vi "Begin.vi"(8 "error in":errorcluster) -> (0 "error out":errorcluster, 2 "pt cluster out":T1={"linear acuator left"={"DeviceStatus"={"status"=FALSE, "code"=0, "source"=""}, "Type"=enum."PWM", "PWM"={"PWM Channel"=enum."Invalid", "DeadBand"={"Name"="", "maxPositivePwm"=0, "minPositivePwm"=0, "centerPwm"=0, "maxNegativePwm"=0, "minNegativePwm"=0, "angularRange"=0}}, "CAN"={"Device Number"=0, "SetOutput VI Ref"=variant(refnum<vi> refnum), "GetOutput VI Ref"=variant(refnum<vi> refnum), "Enable VI Ref"=variant(refnum<vi> refnum), "Disable VI Ref"=variant(refnum<vi> refnum), "Data"=variant}, "Invert"=FALSE, "DIO PWM"={"PWM \"Enable\" Channel"=enum."Invalid", "DIOChannel"=enum."Invalid", "PWM Rate"=0.0}}, "arm extension"={"DeviceStatus"={"status"=FALSE, "code"=0, "source"=""}, "Type"=enum."PWM", "PWM"={"PWM Channel"=enum."Invalid", "DeadBand"={"Name"="", "maxPositivePwm"=0, "minPositivePwm"=0, "centerPwm"=0, "maxNegativePwm"=0, "minNegativePwm"=0, "angularRange"=0}}, "CAN"={"Device Number"=0, "SetOutput VI Ref"=variant(refnum<vi> refnum), "GetOutput VI Ref"=variant(refnum<vi> refnum), "Enable VI Ref"=variant(refnum<vi> refnum), "Disable VI Ref"=variant(refnum<vi> refnum), "Data"=variant}, "Invert"=FALSE, "DIO PWM"={"PWM \"Enable\" Channel"=enum."Invalid", "DIOChannel"=enum."Invalid", "PWM Rate"=0.0}}, "turret"={"DeviceStatus"={"status"=FALSE, "code"=0, "source"=""}, "Type"=enum."PWM", "PWM"={"PWM Channel"=enum."Invalid", "DeadBand"={"Name"="", "maxPositivePwm"=0, "minPositivePwm"=0, "centerPwm"=0, "maxNegativePwm"=0, "minNegativePwm"=0, "angularRange"=0}}, "CAN"={"Device Number"=0, "SetOutput VI Ref"=variant(refnum<vi> refnum), "GetOutput VI Ref"=variant(refnum<vi> refnum), "Enable VI Ref"=variant(refnum<vi> refnum), "Disable VI Ref"=variant(refnum<vi> refnum), "Data"=variant}, "Invert"=FALSE, "DIO PWM"={"PWM \"Enable\" Channel"=enum."Invalid", "DIOChannel"=enum."Invalid", "PWM Rate"=0.0}}, "hood"={"DeviceStatus"={"status"=FALSE, "code"=0, "source"=""}, "Type"=enum."PWM", "PWM"={"PWM Channel"=enum."Invalid", "DeadBand"={"Name"="", "maxPositivePwm"=0, "minPositivePwm"=0, "centerPwm"=0, "maxNegativePwm"=0, "minNegativePwm"=0, "angularRange"=0}}, "CAN"={"Device Number"=0, "SetOutput VI Ref"=variant(refnum<vi> refnum), "GetOutput VI Ref"=variant(refnum<vi> refnum), "Enable VI Ref"=variant(refnum<vi> refnum), "Disable VI Ref"=variant(refnum<vi> refnum), "Data"=variant}, "Invert"=FALSE, "DIO PWM"={"PWM \"Enable\" Channel"=enum."Invalid", "DIOChannel"=enum."Invalid", "PWM Rate"=0.0}}, "climb brake"={"DevStatus"={"status"=FALSE, "code"=0, "source"=""}, "Pneumatics Control Module"=0, "Forward Solenoid Channel"=enum."Solenoid 1", "Reverse Solenoid Channel"=enum."Invalid"}, "buddy climb"={"DevStatus"={"status"=FALSE, "code"=0, "source"=""}, "Pneumatics Control Module"=0, "Forward Solenoid Channel"=enum."Solenoid 1", "Reverse Solenoid Channel"=enum."Invalid"}, "drivetrain shifter"={"DevStatus"={"status"=FALSE, "code"=0, "source"=""}, "Pneumatics Control Module"=0, "Forward Solenoid Channel"=enum."Solenoid 1", "Reverse Solenoid Channel"=enum."Invalid"}, "hood"={"DevStatus"={"status"=FALSE, "code"=0, "source"=""}, "Pneumatics Control Module"=0, "Forward Solenoid Channel"=enum."Solenoid 1", "Reverse Solenoid Channel"=enum."Invalid"}, "climber encoder"={"DevStatus"={"status"=FALSE, "code"=0, "source"=""}, "EncoderIndex"=enum."Enc 0", "CounterIndex"=enum."Ctr 0", "DistancePerCount"=1.0, "Decoding Type"=enum."4x"}, "shooter encoder"={"DevStatus"={"status"=FALSE, "code"=0, "source"=""}, "EncoderIndex"=enum."Enc 0", "CounterIndex"=enum."Ctr 0", "DistancePerCount"=1.0, "Decoding Type"=enum."4x"}, "color sensor"={"I2CDevRef"={"DevStatus"={"status"=FALSE, "code"=0, "source"=""}, "Device Address"=0, "Handle"=0, "I2C Bus"=enum."Invalid"}}, "linear acuator left pot"={"DevStatus"={"status"=FALSE, "code"=0, "source"=""}, "Analog Channel"=enum."Invalid", "Invert Output"=FALSE}, "linear acuator right pot "={"DevStatus"={"status"=FALSE, "code"=0, "source"=""}, "Analog Channel"=enum."Invalid", "Invert Output"=FALSE}, "auto balancer pot"={"DevStatus"={"status"=FALSE, "code"=0, "source"=""}, "Analog Channel"=enum."Invalid", "Invert Output"=FALSE}, "shooter"={"DeviceStatus"={"status"=FALSE, "code"=0, "source"=""}, "Type"=enum."PWM", "PWM"={"PWM Channel"=enum."Invalid", "DeadBand"={"Name"="", "maxPositivePwm"=0, "minPositivePwm"=0, "centerPwm"=0, "maxNegativePwm"=0, "minNegativePwm"=0, "angularRange"=0}}, "CAN"={"Device Number"=0, "SetOutput VI Ref"=variant(refnum<vi> refnum), "GetOutput VI Ref"=variant(refnum<vi> refnum), "Enable VI Ref"=variant(refnum<vi> refnum), "Disable VI Ref"=variant(refnum<vi> refnum), "Data"=variant}, "Invert"=FALSE, "DIO PWM"={"PWM \"Enable\" Channel"=enum."Invalid", "DIOChannel"=enum."Invalid", "PWM Rate"=0.0}}, "hopper"={"DeviceStatus"={"status"=FALSE, "code"=0, "source"=""}, "Type"=enum."PWM", "PWM"={"PWM Channel"=enum."Invalid", "DeadBand"={"Name"="", "maxPositivePwm"=0, "minPositivePwm"=0, "centerPwm"=0, "maxNegativePwm"=0, "minNegativePwm"=0, "angularRange"=0}}, "CAN"={"Device Number"=0, "SetOutput VI Ref"=variant(refnum<vi> refnum), "GetOutput VI Ref"=variant(refnum<vi> refnum), "Enable VI Ref"=variant(refnum<vi> refnum), "Disable VI Ref"=variant(refnum<vi> refnum), "Data"=variant}, "Invert"=FALSE, "DIO PWM"={"PWM \"Enable\" Channel"=enum."Invalid", "DIOChannel"=enum."Invalid", "PWM Rate"=0.0}}, "feeder"={"DeviceStatus"={"status"=FALSE, "code"=0, "source"=""}, "Type"=enum."PWM", "PWM"={"PWM Channel"=enum."Invalid", "DeadBand"={"Name"="", "maxPositivePwm"=0, "minPositivePwm"=0, "centerPwm"=0, "maxNegativePwm"=0, "minNegativePwm"=0, "angularRange"=0}}, "CAN"={"Device Number"=0, "SetOutput VI Ref"=variant(refnum<vi> refnum), "GetOutput VI Ref"=variant(refnum<vi> refnum), "Enable VI Ref"=variant(refnum<vi> refnum), "Disable VI Ref"=variant(refnum<vi> refnum), "Data"=variant}, "Invert"=FALSE, "DIO PWM"={"PWM \"Enable\" Channel"=enum."Invalid", "DIOChannel"=enum."Invalid", "PWM Rate"=0.0}}, "intake"={"DeviceStatus"={"status"=FALSE, "code"=0, "source"=""}, "Type"=enum."PWM", "PWM"={"PWM Channel"=enum."Invalid", "DeadBand"={"Name"="", "maxPositivePwm"=0, "minPositivePwm"=0, "centerPwm"=0, "maxNegativePwm"=0, "minNegativePwm"=0, "angularRange"=0}}, "CAN"={"Device Number"=0, "SetOutput VI Ref"=variant(refnum<vi> refnum), "GetOutput VI Ref"=variant(refnum<vi> refnum), "Enable VI Ref"=variant(refnum<vi> refnum), "Disable VI Ref"=variant(refnum<vi> refnum), "Data"=variant}, "Invert"=FALSE, "DIO PWM"={"PWM \"Enable\" Channel"=enum."Invalid", "DIOChannel"=enum."Invalid", "PWM Rate"=0.0}}, "auto balance"={"DeviceStatus"={"status"=FALSE, "code"=0, "source"=""}, "Type"=enum."PWM", "PWM"={"PWM Channel"=enum."Invalid", "DeadBand"={"Name"="", "maxPositivePwm"=0, "minPositivePwm"=0, "centerPwm"=0, "maxNegativePwm"=0, "minNegativePwm"=0, "angularRange"=0}}, "CAN"={"Device Number"=0, "SetOutput VI Ref"=variant(refnum<vi> refnum), "GetOutput VI Ref"=variant(refnum<vi> refnum), "Enable VI Ref"=variant(refnum<vi> refnum), "Disable VI Ref"=variant(refnum<vi> refnum), "Data"=variant}, "Invert"=FALSE, "DIO PWM"={"PWM \"Enable\" Channel"=enum."Invalid", "DIOChannel"=enum."Invalid", "PWM Rate"=0.0}}, "linear acuator right"={"DeviceStatus"={"status"=FALSE, "code"=0, "source"=""}, "Type"=enum."PWM", "PWM"={"PWM Channel"=enum."Invalid", "DeadBand"={"Name"="", "maxPositivePwm"=0, "minPositivePwm"=0, "centerPwm"=0, "maxNegativePwm"=0, "minNegativePwm"=0, "angularRange"=0}}, "CAN"={"Device Number"=0, "SetOutput VI Ref"=variant(refnum<vi> refnum), "GetOutput VI Ref"=variant(refnum<vi> refnum), "Enable VI Ref"=variant(refnum<vi> refnum), "Disable VI Ref"=variant(refnum<vi> refnum), "Data"=variant}, "Invert"=FALSE, "DIO PWM"={"PWM \"Enable\" Channel"=enum."Invalid", "DIOChannel"=enum."Invalid", "PWM Rate"=0.0}}} {"color sensor"."I2CDevRef"."Device Address" format="%.0x"}, 3 "Teleop/Auto Cluster Out":T18={"x Joystick"={"Device"=enum."USB 1"}, "y Joystick"={"Device"=enum."USB 1"}, "controller"={"Device"=enum."USB 1"}, "right drive encoder"={"DevStatus"={"status"=FALSE, "code"=0, "source"=""}, "EncoderIndex"=enum."Enc 0", "CounterIndex"=enum."Ctr 0", "DistancePerCount"=1.0, "Decoding Type"=enum."4x"}, "left drive encoder"={"DevStatus"={"status"=FALSE, "code"=0, "source"=""}, "EncoderIndex"=enum."Enc 0", "CounterIndex"=enum."Ctr 0", "DistancePerCount"=1.0, "Decoding Type"=enum."4x"}, "drive motors"={"DevStatus"={"status"=FALSE, "code"=0, "source"=""}, "Motors[]"=[], "Square Inputs"=FALSE, "Max Output"=1.0}, "gyro"={"DeviceStatus"={"status"=FALSE, "code"=0, "source"=""}, "Device Number"=0, "Type"=352321536, "Device ID"=0, "Handle"=0, "UsageFrame"=0, "Library Path"=path ""}, "drive buttons"={"Device"=enum."USB 1"}} {"gyro"."Type" items=["CAN"=352321536, "TalonSRX"=33554432]})   [LabVIEW 2019]
doc: "Called before other user functions, this VI is expected to open initial I/O refnums, load in file data, and do all program initialization. Notice that the <B>error out</B> terminal is simply used for data flow. Wiring it to other structures or subVIs ensures that this VI runs first."
uses:
  <vilib>/Rock Robotics/WPI/RobotDrive/WPI_RobotDriveDevRef.ctl
  <vilib>/Rock Robotics/WPI/MotorControl/WPI_MotorControlDeviceRef.ctl
  <vilib>/Rock Robotics/WPI/MotorControl/WPI_MotorControlType.ctl
  <vilib>/Rock Robotics/SystemInterfaces/DIO/FPGA_DIOPWMChannel.ctl
  <vilib>/Rock Robotics/WPI/PWM/WPI_PWMDeadband.ctl
  <vilib>/Rock Robotics/SystemInterfaces/DIO/FPGA_DIOChannel.ctl
  teleop auto cluster.ctl
  <vilib>/Rock Robotics/WPI/Joystick/WPI_JoystickDevRef.ctl
  <vilib>/Rock Robotics/WPI/Joystick/WPI_JoystickDeviceEnum.ctl
  <vilib>/Rock Robotics/WPI/Encoder/WPI_EncoderDevRef.ctl
  <vilib>/Rock Robotics/SystemInterfaces/Encoder/FPGA_EncoderIdx.ctl
  <vilib>/Rock Robotics/SystemInterfaces/Counter/FPGA_CounterCtrSystemIndex.ctl
  <vilib>/Rock Robotics/WPI/Encoder/WPI_EncoderType.ctl
  <vilib>/Rock Robotics/WPI/ThirdParty/Phoenix-LabVIEW/Pigeon IMU/CTRE_PigeonIMU_DeviceRef.ctl
  <vilib>/Rock Robotics/WPI/ThirdParty/Phoenix-LabVIEW/Pigeon IMU/CTRE_PigeonIMU_ConnectionType.ctl
  ptclustergood.ctl
  <vilib>/Rock Robotics/WPI/Solenoid/WPI_SolenoidDevRef.ctl
  <vilib>/Rock Robotics/WPI/Solenoid/WPI_SolenoidChannel.ctl
  <vilib>/Rock Robotics/WPI/ThirdParty/REV Robotics/Color SensorV3/Typedef/Color Sensor V3 DevRef.ctl
  <vilib>/Rock Robotics/WPI/I2C/WPI_I2CDevRef.ctl
  <vilib>/Rock Robotics/SystemInterfaces/i2clib/i2c_bus.ctl
  <vilib>/Rock Robotics/WPI/Potentiometer/WPI_PotentiometerDevRef.ctl
  <vilib>/Rock Robotics/SystemInterfaces/AI/FPGA_AIChannel.ctl
  <vilib>/Rock Robotics/WPI/DriverStation/WPI_DriverStationRobotMode2.ctl
  <vilib>/Rock Robotics/WPI/Solenoid/WPI_SolenoidValue.ctl
  <vilib>/Rock Robotics/WPI/ThirdParty/Phoenix-LabVIEW/Pigeon IMU/CTRE_PigeonIMU_TareType.ctl
  Robot Global Data.vi
  <vilib>/Rock Robotics/WPI/Counter/WPI_CounterDigitalInputToDigitalSource.vi
  <vilib>/Rock Robotics/WPI/Solenoid/WPI_SolenoidOpenDouble.vi
  <vilib>/Rock Robotics/WPI/Solenoid/WPI_SolenoidSetEnum.vi
  <vilib>/Rock Robotics/WPI/ThirdParty/Phoenix-LabVIEW/Pigeon IMU/CTRE_PigeonIMU_Open_CAN.vi
  GlobalVariables.vi
panel:
  in  "pt cluster":T1={"linear acuator left"={"DeviceStatus"={"status"=FALSE, "code"=0, "source"=""}, "Type"=enum."PWM", "PWM"={"PWM Channel"=enum."Invalid", "DeadBand"={"Name"="", "maxPositivePwm"=0, "minPositivePwm"=0, "centerPwm"=0, "maxNegativePwm"=0, "minNegativePwm"=0, "angularRange"=0}}, "CAN"={"Device Number"=0, "SetOutput VI Ref"=variant(refnum<vi> refnum), "GetOutput VI Ref"=variant(refnum<vi> refnum), "Enable VI Ref"=variant(refnum<vi> refnum), "Disable VI Ref"=variant(refnum<vi> refnum), "Data"=variant}, "Invert"=FALSE, "DIO PWM"={"PWM \"Enable\" Channel"=enum."Invalid", "DIOChannel"=enum."Invalid", "PWM Rate"=0.0}}, "arm extension"={"DeviceStatus"={"status"=FALSE, "code"=0, "source"=""}, "Type"=enum."PWM", "PWM"={"PWM Channel"=enum."Invalid", "DeadBand"={"Name"="", "maxPositivePwm"=0, "minPositivePwm"=0, "centerPwm"=0, "maxNegativePwm"=0, "minNegativePwm"=0, "angularRange"=0}}, "CAN"={"Device Number"=0, "SetOutput VI Ref"=variant(refnum<vi> refnum), "GetOutput VI Ref"=variant(refnum<vi> refnum), "Enable VI Ref"=variant(refnum<vi> refnum), "Disable VI Ref"=variant(refnum<vi> refnum), "Data"=variant}, "Invert"=FALSE, "DIO PWM"={"PWM \"Enable\" Channel"=enum."Invalid", "DIOChannel"=enum."Invalid", "PWM Rate"=0.0}}, "turret"={"DeviceStatus"={"status"=FALSE, "code"=0, "source"=""}, "Type"=enum."PWM", "PWM"={"PWM Channel"=enum."Invalid", "DeadBand"={"Name"="", "maxPositivePwm"=0, "minPositivePwm"=0, "centerPwm"=0, "maxNegativePwm"=0, "minNegativePwm"=0, "angularRange"=0}}, "CAN"={"Device Number"=0, "SetOutput VI Ref"=variant(refnum<vi> refnum), "GetOutput VI Ref"=variant(refnum<vi> refnum), "Enable VI Ref"=variant(refnum<vi> refnum), "Disable VI Ref"=variant(refnum<vi> refnum), "Data"=variant}, "Invert"=FALSE, "DIO PWM"={"PWM \"Enable\" Channel"=enum."Invalid", "DIOChannel"=enum."Invalid", "PWM Rate"=0.0}}, "hood"={"DeviceStatus"={"status"=FALSE, "code"=0, "source"=""}, "Type"=enum."PWM", "PWM"={"PWM Channel"=enum."Invalid", "DeadBand"={"Name"="", "maxPositivePwm"=0, "minPositivePwm"=0, "centerPwm"=0, "maxNegativePwm"=0, "minNegativePwm"=0, "angularRange"=0}}, "CAN"={"Device Number"=0, "SetOutput VI Ref"=variant(refnum<vi> refnum), "GetOutput VI Ref"=variant(refnum<vi> refnum), "Enable VI Ref"=variant(refnum<vi> refnum), "Disable VI Ref"=variant(refnum<vi> refnum), "Data"=variant}, "Invert"=FALSE, "DIO PWM"={"PWM \"Enable\" Channel"=enum."Invalid", "DIOChannel"=enum."Invalid", "PWM Rate"=0.0}}, "climb brake"={"DevStatus"={"status"=FALSE, "code"=0, "source"=""}, "Pneumatics Control Module"=0, "Forward Solenoid Channel"=enum."Solenoid 1", "Reverse Solenoid Channel"=enum."Invalid"}, "buddy climb"={"DevStatus"={"status"=FALSE, "code"=0, "source"=""}, "Pneumatics Control Module"=0, "Forward Solenoid Channel"=enum."Solenoid 1", "Reverse Solenoid Channel"=enum."Invalid"}, "drivetrain shifter"={"DevStatus"={"status"=FALSE, "code"=0, "source"=""}, "Pneumatics Control Module"=0, "Forward Solenoid Channel"=enum."Solenoid 1", "Reverse Solenoid Channel"=enum."Invalid"}, "hood"={"DevStatus"={"status"=FALSE, "code"=0, "source"=""}, "Pneumatics Control Module"=0, "Forward Solenoid Channel"=enum."Solenoid 1", "Reverse Solenoid Channel"=enum."Invalid"}, "climber encoder"={"DevStatus"={"status"=FALSE, "code"=0, "source"=""}, "EncoderIndex"=enum."Enc 0", "CounterIndex"=enum."Ctr 0", "DistancePerCount"=1.0, "Decoding Type"=enum."4x"}, "shooter encoder"={"DevStatus"={"status"=FALSE, "code"=0, "source"=""}, "EncoderIndex"=enum."Enc 0", "CounterIndex"=enum."Ctr 0", "DistancePerCount"=1.0, "Decoding Type"=enum."4x"}, "color sensor"={"I2CDevRef"={"DevStatus"={"status"=FALSE, "code"=0, "source"=""}, "Device Address"=0, "Handle"=0, "I2C Bus"=enum."Invalid"}}, "linear acuator left pot"={"DevStatus"={"status"=FALSE, "code"=0, "source"=""}, "Analog Channel"=enum."Invalid", "Invert Output"=FALSE}, "linear acuator right pot "={"DevStatus"={"status"=FALSE, "code"=0, "source"=""}, "Analog Channel"=enum."Invalid", "Invert Output"=FALSE}, "auto balancer pot"={"DevStatus"={"status"=FALSE, "code"=0, "source"=""}, "Analog Channel"=enum."Invalid", "Invert Output"=FALSE}, "shooter"={"DeviceStatus"={"status"=FALSE, "code"=0, "source"=""}, "Type"=enum."PWM", "PWM"={"PWM Channel"=enum."Invalid", "DeadBand"={"Name"="", "maxPositivePwm"=0, "minPositivePwm"=0, "centerPwm"=0, "maxNegativePwm"=0, "minNegativePwm"=0, "angularRange"=0}}, "CAN"={"Device Number"=0, "SetOutput VI Ref"=variant(refnum<vi> refnum), "GetOutput VI Ref"=variant(refnum<vi> refnum), "Enable VI Ref"=variant(refnum<vi> refnum), "Disable VI Ref"=variant(refnum<vi> refnum), "Data"=variant}, "Invert"=FALSE, "DIO PWM"={"PWM \"Enable\" Channel"=enum."Invalid", "DIOChannel"=enum."Invalid", "PWM Rate"=0.0}}, "hopper"={"DeviceStatus"={"status"=FALSE, "code"=0, "source"=""}, "Type"=enum."PWM", "PWM"={"PWM Channel"=enum."Invalid", "DeadBand"={"Name"="", "maxPositivePwm"=0, "minPositivePwm"=0, "centerPwm"=0, "maxNegativePwm"=0, "minNegativePwm"=0, "angularRange"=0}}, "CAN"={"Device Number"=0, "SetOutput VI Ref"=variant(refnum<vi> refnum), "GetOutput VI Ref"=variant(refnum<vi> refnum), "Enable VI Ref"=variant(refnum<vi> refnum), "Disable VI Ref"=variant(refnum<vi> refnum), "Data"=variant}, "Invert"=FALSE, "DIO PWM"={"PWM \"Enable\" Channel"=enum."Invalid", "DIOChannel"=enum."Invalid", "PWM Rate"=0.0}}, "feeder"={"DeviceStatus"={"status"=FALSE, "code"=0, "source"=""}, "Type"=enum."PWM", "PWM"={"PWM Channel"=enum."Invalid", "DeadBand"={"Name"="", "maxPositivePwm"=0, "minPositivePwm"=0, "centerPwm"=0, "maxNegativePwm"=0, "minNegativePwm"=0, "angularRange"=0}}, "CAN"={"Device Number"=0, "SetOutput VI Ref"=variant(refnum<vi> refnum), "GetOutput VI Ref"=variant(refnum<vi> refnum), "Enable VI Ref"=variant(refnum<vi> refnum), "Disable VI Ref"=variant(refnum<vi> refnum), "Data"=variant}, "Invert"=FALSE, "DIO PWM"={"PWM \"Enable\" Channel"=enum."Invalid", "DIOChannel"=enum."Invalid", "PWM Rate"=0.0}}, "intake"={"DeviceStatus"={"status"=FALSE, "code"=0, "source"=""}, "Type"=enum."PWM", "PWM"={"PWM Channel"=enum."Invalid", "DeadBand"={"Name"="", "maxPositivePwm"=0, "minPositivePwm"=0, "centerPwm"=0, "maxNegativePwm"=0, "minNegativePwm"=0, "angularRange"=0}}, "CAN"={"Device Number"=0, "SetOutput VI Ref"=variant(refnum<vi> refnum), "GetOutput VI Ref"=variant(refnum<vi> refnum), "Enable VI Ref"=variant(refnum<vi> refnum), "Disable VI Ref"=variant(refnum<vi> refnum), "Data"=variant}, "Invert"=FALSE, "DIO PWM"={"PWM \"Enable\" Channel"=enum."Invalid", "DIOChannel"=enum."Invalid", "PWM Rate"=0.0}}, "auto balance"={"DeviceStatus"={"status"=FALSE, "code"=0, "source"=""}, "Type"=enum."PWM", "PWM"={"PWM Channel"=enum."Invalid", "DeadBand"={"Name"="", "maxPositivePwm"=0, "minPositivePwm"=0, "centerPwm"=0, "maxNegativePwm"=0, "minNegativePwm"=0, "angularRange"=0}}, "CAN"={"Device Number"=0, "SetOutput VI Ref"=variant(refnum<vi> refnum), "GetOutput VI Ref"=variant(refnum<vi> refnum), "Enable VI Ref"=variant(refnum<vi> refnum), "Disable VI Ref"=variant(refnum<vi> refnum), "Data"=variant}, "Invert"=FALSE, "DIO PWM"={"PWM \"Enable\" Channel"=enum."Invalid", "DIOChannel"=enum."Invalid", "PWM Rate"=0.0}}, "linear acuator right"={"DeviceStatus"={"status"=FALSE, "code"=0, "source"=""}, "Type"=enum."PWM", "PWM"={"PWM Channel"=enum."Invalid", "DeadBand"={"Name"="", "maxPositivePwm"=0, "minPositivePwm"=0, "centerPwm"=0, "maxNegativePwm"=0, "minNegativePwm"=0, "angularRange"=0}}, "CAN"={"Device Number"=0, "SetOutput VI Ref"=variant(refnum<vi> refnum), "GetOutput VI Ref"=variant(refnum<vi> refnum), "Enable VI Ref"=variant(refnum<vi> refnum), "Disable VI Ref"=variant(refnum<vi> refnum), "Data"=variant}, "Invert"=FALSE, "DIO PWM"={"PWM \"Enable\" Channel"=enum."Invalid", "DIOChannel"=enum."Invalid", "PWM Rate"=0.0}}} {"color sensor"."I2CDevRef"."Device Address" format="%.0x"}
  in  "Teleop/Auto Cluster":T18={"x Joystick"={"Device"=enum."USB 1"}, "y Joystick"={"Device"=enum."USB 1"}, "controller"={"Device"=enum."USB 1"}, "right drive encoder"={"DevStatus"={"status"=FALSE, "code"=0, "source"=""}, "EncoderIndex"=enum."Enc 0", "CounterIndex"=enum."Ctr 0", "DistancePerCount"=1.0, "Decoding Type"=enum."4x"}, "left drive encoder"={"DevStatus"={"status"=FALSE, "code"=0, "source"=""}, "EncoderIndex"=enum."Enc 0", "CounterIndex"=enum."Ctr 0", "DistancePerCount"=1.0, "Decoding Type"=enum."4x"}, "drive motors"={"DevStatus"={"status"=FALSE, "code"=0, "source"=""}, "Motors[]"=[], "Square Inputs"=FALSE, "Max Output"=1.0}, "gyro"={"DeviceStatus"={"status"=FALSE, "code"=0, "source"=""}, "Device Number"=0, "Type"=352321536, "Device ID"=0, "Handle"=0, "UsageFrame"=0, "Library Path"=path ""}, "drive buttons"={"Device"=enum."USB 1"}} {"gyro"."Type" items=["CAN"=352321536, "TalonSRX"=33554432]}
  in  "RobotDriveDevRef":T21={"DevStatus"={"status"=FALSE, "code"=0, "source"=""}, "Motors[]"=[], "Square Inputs"=FALSE, "Max Output"=1.0}
  in  "DevStatus":errorcluster
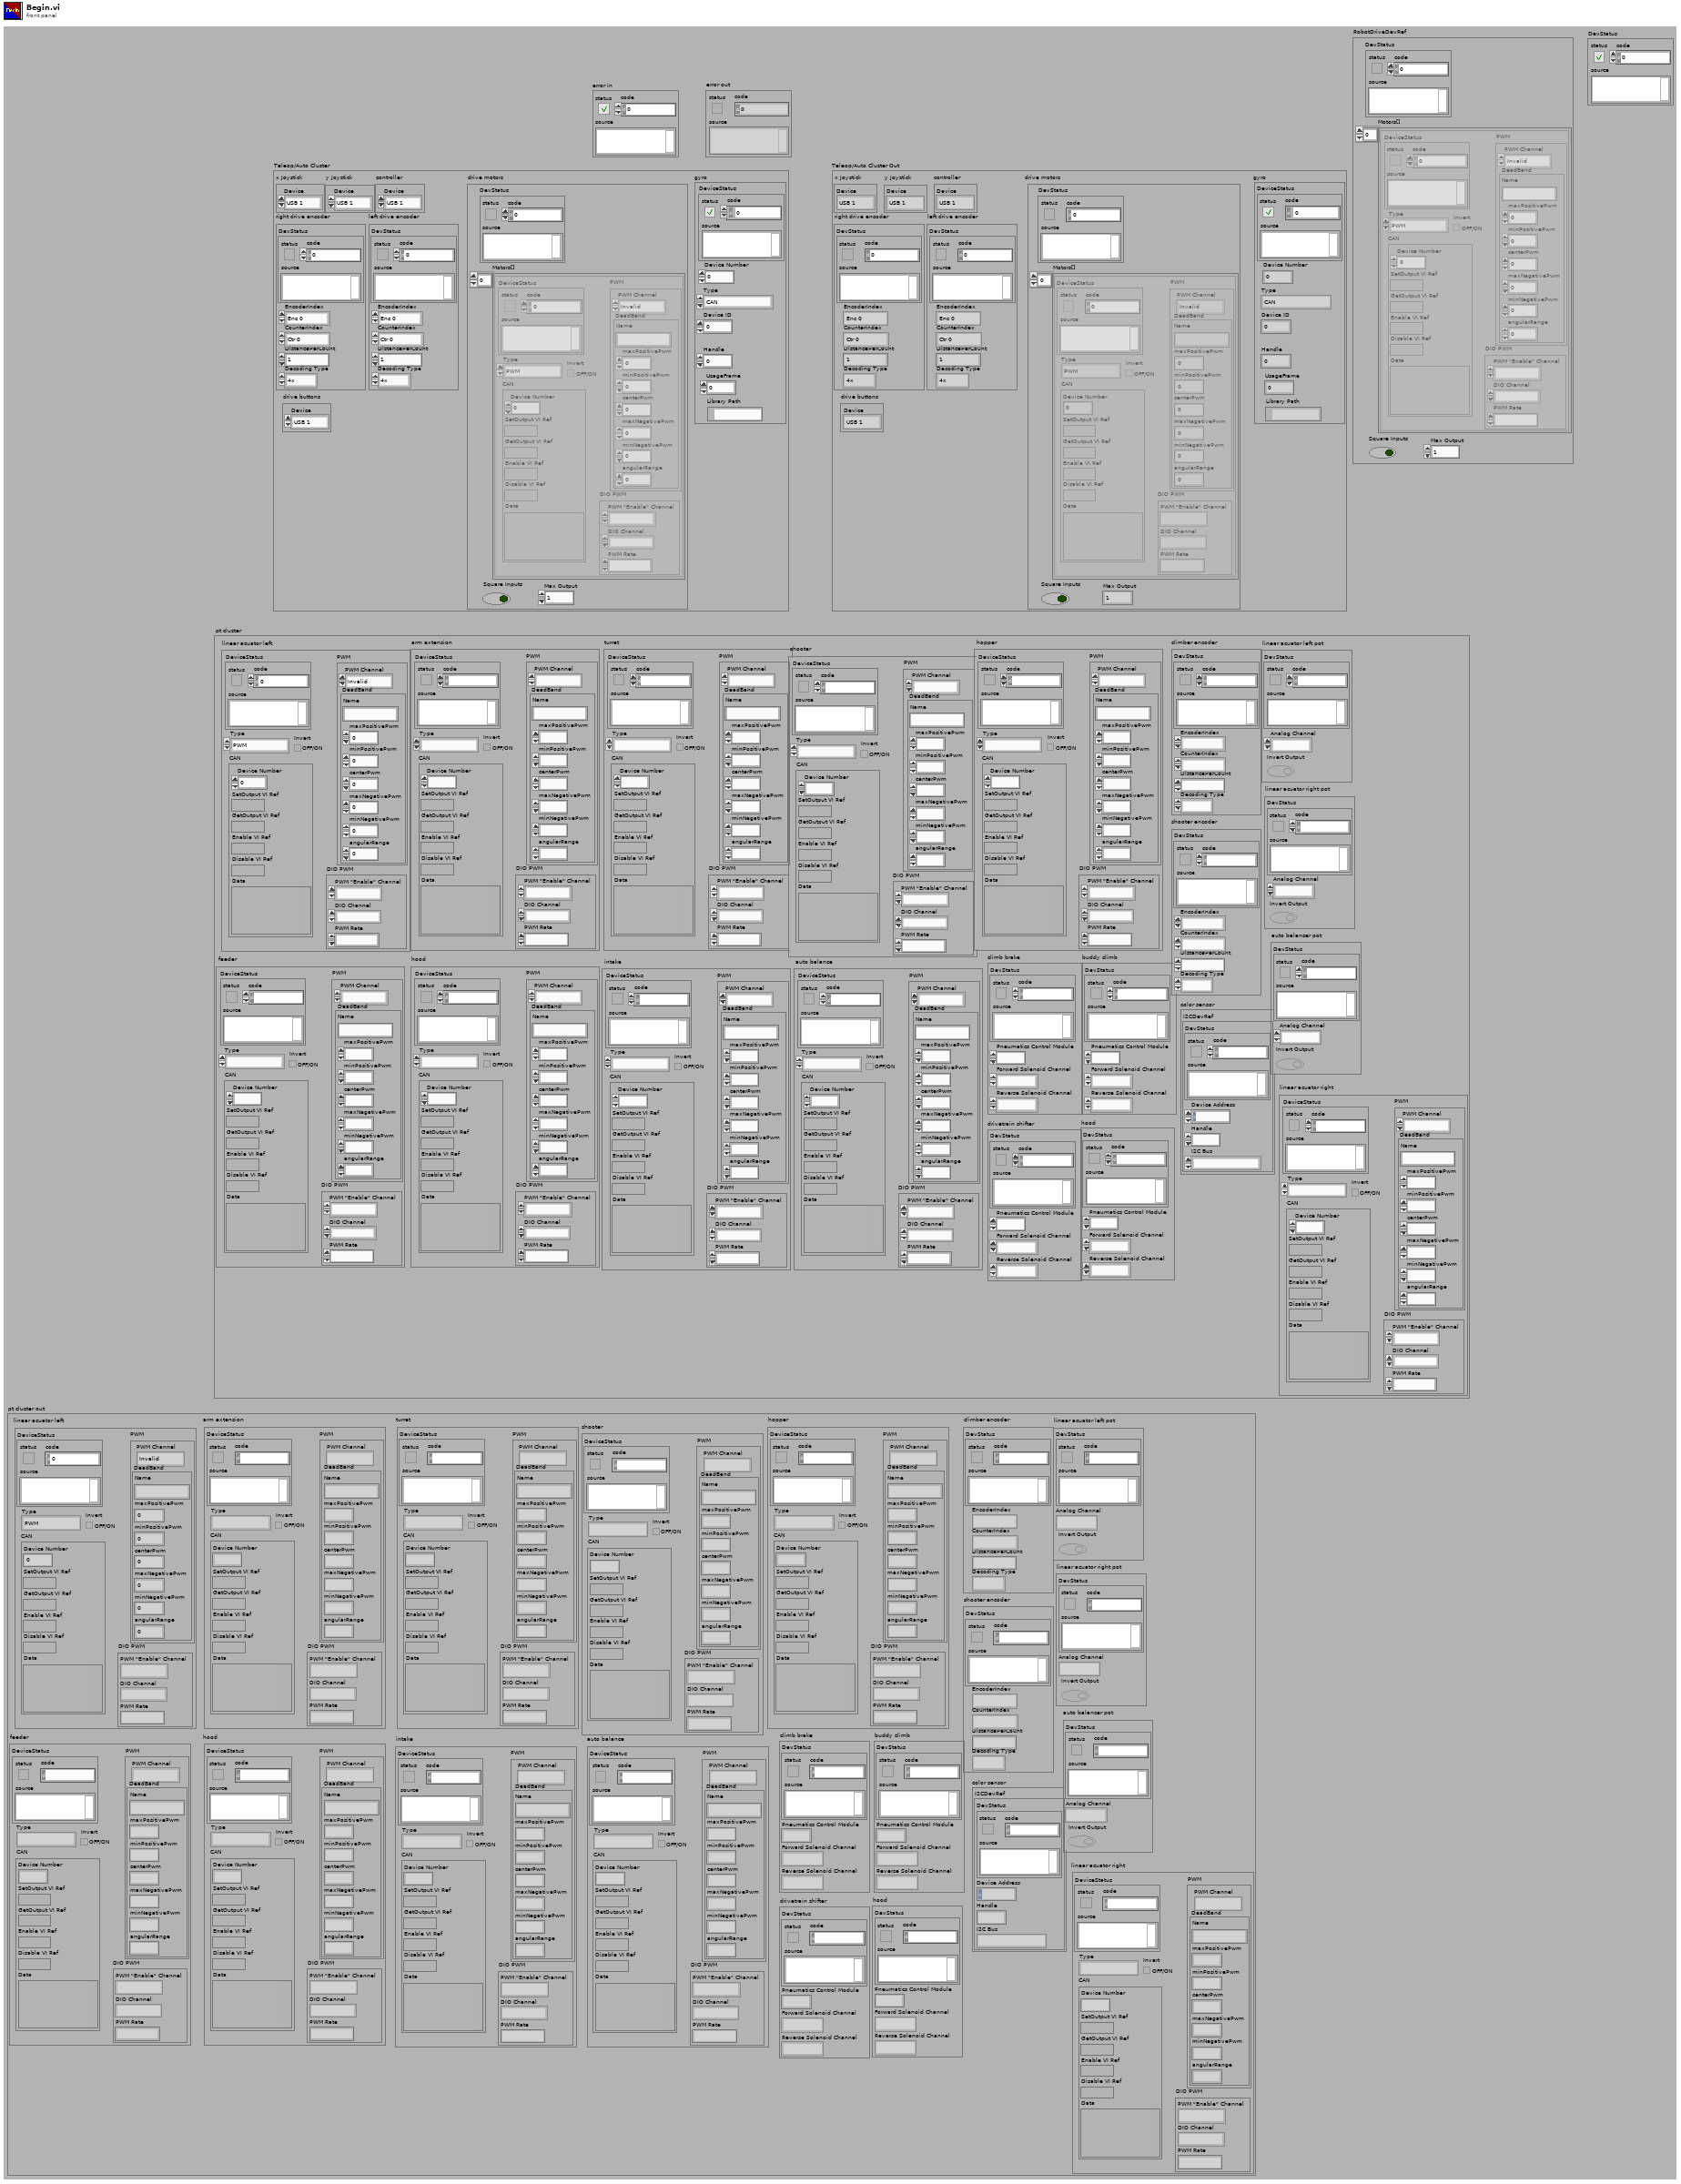
[diagram p1: front panel]
types:
  T1 = typedef "ptclustergood.ctl" = cluster{"linear acuator left":T2, "arm extension":T2, "turret":T2, "hood":T2, "climb brake":T7, "buddy climb":T7, "drivetrain shifter":T7, "hood":T7, "climber encoder":T9, "shooter encoder":T9, "color sensor":T13, "linear acuator left pot":T16, "linear acuator right pot ":T16, "auto balancer pot":T16, "shooter":T2, "hopper":T2, "feeder":T2, "intake":T2, "auto balance":T2, "linear acuator right":T2}
  T2 = typedef "WPI_MotorControlDeviceRef.ctl" = cluster{"DeviceStatus":errorcluster, "Type":T3, "PWM":cluster{"PWM Channel":T4, "DeadBand":T5}, "CAN":cluster{"Device Number":u8, "SetOutput VI Ref":variant, "GetOutput VI Ref":variant, "Enable VI Ref":variant, "Disable VI Ref":variant, "Data":variant}, "Invert":bool, "DIO PWM":cluster{"PWM \"Enable\" Channel":T4, "DIOChannel":T6, "PWM Rate":dbl}}
  T3 = typedef "WPI_MotorControlType.ctl" = enum16{"PWM", "CAN", "DIO PWM"}
  T4 = typedef "FPGA_DIOPWMChannel.ctl" = enum8{"PWM 0", "PWM 1", "PWM 2", "PWM 3", "PWM 4", "PWM 5", "PWM 6", "PWM 7", "PWM 8", "PWM 9", "PWM MXP 0", "PWM MXP 1", "PWM MXP 2", "PWM MXP 3", "PWM MXP 4", "PWM MXP 5", "PWM MXP 6", "PWM MXP 7", "PWM MXP 8", "PWM MXP 9", "Invalid"}
  T5 = typedef "WPI_PWMDeadband.ctl" = cluster{"Name":string, "maxPositivePwm":i32, "minPositivePwm":i32, "centerPwm":i32, "maxNegativePwm":i32, "minNegativePwm":i32, "angularRange":u16}
  T6 = typedef "FPGA_DIOChannel.ctl" = enum8{"DIO 0", "DIO 1", "DIO 2", "DIO 3", "DIO 4", "DIO 5", "DIO 6", "DIO 7", "DIO 8", "DIO 9", "DIO MXP 0", "DIO MXP 1", "DIO MXP 2", "DIO MXP 3", "DIO MXP 4", "DIO MXP 5", "DIO MXP 6", "DIO MXP 7", "DIO MXP 8", "DIO MXP 9", "DIO MXP 10", "DIO MXP 11", "DIO MXP 12", "DIO MXP 13", "DIO MXP 14", "DIO MXP 15", "SPI Port CS1", "SPI Port CS2", "SPI Port CS3", "SPI Port MISO", "SPI Port MOSI", "Invalid"}
  T7 = typedef "WPI_SolenoidDevRef.ctl" = cluster{"DevStatus":errorcluster, "Pneumatics Control Module":u8, "Forward Solenoid Channel":T8, "Reverse Solenoid Channel":T8}
  T8 = typedef "WPI_SolenoidChannel.ctl" = enum8{"Solenoid 0", "Solenoid 1", "Solenoid 2", "Solenoid 3", "Solenoid 4", "Solenoid 5", "Solenoid 6", "Solenoid 7", "Invalid"}
  T9 = typedef "WPI_EncoderDevRef.ctl" = cluster{"DevStatus":errorcluster, "EncoderIndex":T10, "CounterIndex":T11, "DistancePerCount":dbl, "Decoding Type":T12}
  T10 = typedef "FPGA_EncoderIdx.ctl" = enum8{"Enc 0", "Enc 1", "Enc 2", "Enc 3", "Enc 4", "Enc 5", "Enc 6", "Enc 7", "Invalid"}
  T11 = typedef "FPGA_CounterCtrSystemIndex.ctl" = enum8{"Ctr 0", "Ctr 1", "Ctr 2", "Ctr 3", "Ctr 4", "Ctr 5", "Ctr 6", "Ctr 7", "Invalid"}
  T12 = typedef "WPI_EncoderType.ctl" = enum16{"1x", "2x", "4x"}
  T13 = typedef "Color Sensor V3 DevRef.ctl" = cluster{"I2CDevRef":T14}
  T14 = typedef "WPI_I2CDevRef.ctl" = cluster{"DevStatus":errorcluster, "Device Address":u8, "Handle":i32, "I2C Bus":T15}
  T15 = typedef "i2c_bus.ctl" = enum16{"I2C On-Board", "I2C MXP", "Invalid"}
  T16 = typedef "WPI_PotentiometerDevRef.ctl" = cluster{"DevStatus":errorcluster, "Analog Channel":T17, "Invert Output":bool}
  T17 = typedef "FPGA_AIChannel.ctl" = enum8{"AI 0", "AI 1", "AI 2", "AI 3", "AI MXP 0", "AI MXP 1", "AI MXP 2", "AI MXP 3", "Invalid"}
  T18 = typedef "teleop auto cluster.ctl" = cluster{"x Joystick":T19, "y Joystick":T19, "controller":T19, "right drive encoder":T9, "left drive encoder":T9, "drive motors":T21, "gyro":T22, "drive buttons":T19}
  T19 = typedef "WPI_JoystickDevRef.ctl" = cluster{"Device":T20}
  T20 = typedef "WPI_JoystickDeviceEnum.ctl" = enum16{"USB 0", "USB 1", "USB 2", "USB 3", "USB 4", "USB 5"}
  T21 = typedef "WPI_RobotDriveDevRef.ctl" = cluster{"DevStatus":errorcluster, "Motors[]":T2[], "Square Inputs":bool, "Max Output":dbl}
  T22 = typedef "CTRE_PigeonIMU_DeviceRef.ctl" = cluster{"DeviceStatus":errorcluster, "Device Number":u8, "Type":T23, "Device ID":u32, "Handle":u64, "UsageFrame":u32, "Library Path":path}
  T23 = typedef "CTRE_PigeonIMU_ConnectionType.ctl" = u32
  T24 = enum16{"ground protect", "ground pickup", "control panel", "shooting", "climb", "unjam", "intake shoot"}
  T25 = typedef "WPI_SolenoidValue.ctl" = enum16{"Off", "On", "Forward", "Reverse"}
  T26 = typedef "CTRE_PigeonIMU_TareType.ctl" = u8
  T27 = typedef "WPI_DriverStationRobotMode2.ctl" = enum16{"Autonomous Disabled", "Autonomous Enabled", "Teleop Disabled", "Teleop Enabled", "Disconnected", "Finish", "Test Disabled", "Test Enabled", "Emergency Stopped"}
  T28 = typedef "WPI_DigitalInputDevRef.ctl" = cluster{"DevStatus":errorcluster, "DIO Channel":T6}
  T29 = typedef "FPGA_CounterEncoderSourceConvertionLVSourceType.ctl" = cluster{"DevStatus":errorcluster, "AnalogTriggerMode?":bool, "DigitalMode":cluster{"DIO Channel":T30}, "AnalogTriggerMode":cluster{"AnalogTriggerIndex":T31, "OutputType":T32}}
  T30 = typedef "FPGA_DIODigitalSourceChannel.ctl" = enum8{"DIO 0", "DIO 1", "DIO 2", "DIO 3", "DIO 4", "DIO 5", "DIO 6", "DIO 7", "DIO 8", "DIO 9", "DIO MXP 0", "DIO MXP 1", "DIO MXP 2", "DIO MXP 3", "DIO MXP 4", "DIO MXP 5", "DIO MXP 6", "DIO MXP 7", "DIO MXP 8", "DIO MXP 9", "DIO MXP 10", "DIO MXP 11", "DIO MXP 12", "DIO MXP 13", "DIO MXP 14", "DIO MXP 15", "SPI Port CS1", "SPI Port CS2", "SPI Port CS3", "SPI Port MISO", "SPI Port MOSI", "Disabled"}
  T31 = typedef "FPGA_AnalogTriggerIndex.ctl" = enum8{"Trig 0", "Trig 1", "Trig 2", "Trig 3", "Trig 4", "Trig 5", "Trig 6", "Trig 7", "Invalid"}
  T32 = typedef "FPGA_AnalogTriggerOutType.ctl" = enum16{"InWindow", "TriggerState", "Rising", "Falling"}
  T33 = typedef "WPI_AnalogChannelDevRef.ctl" = cluster{"DevStatus":errorcluster, "Analog Channel":T17}
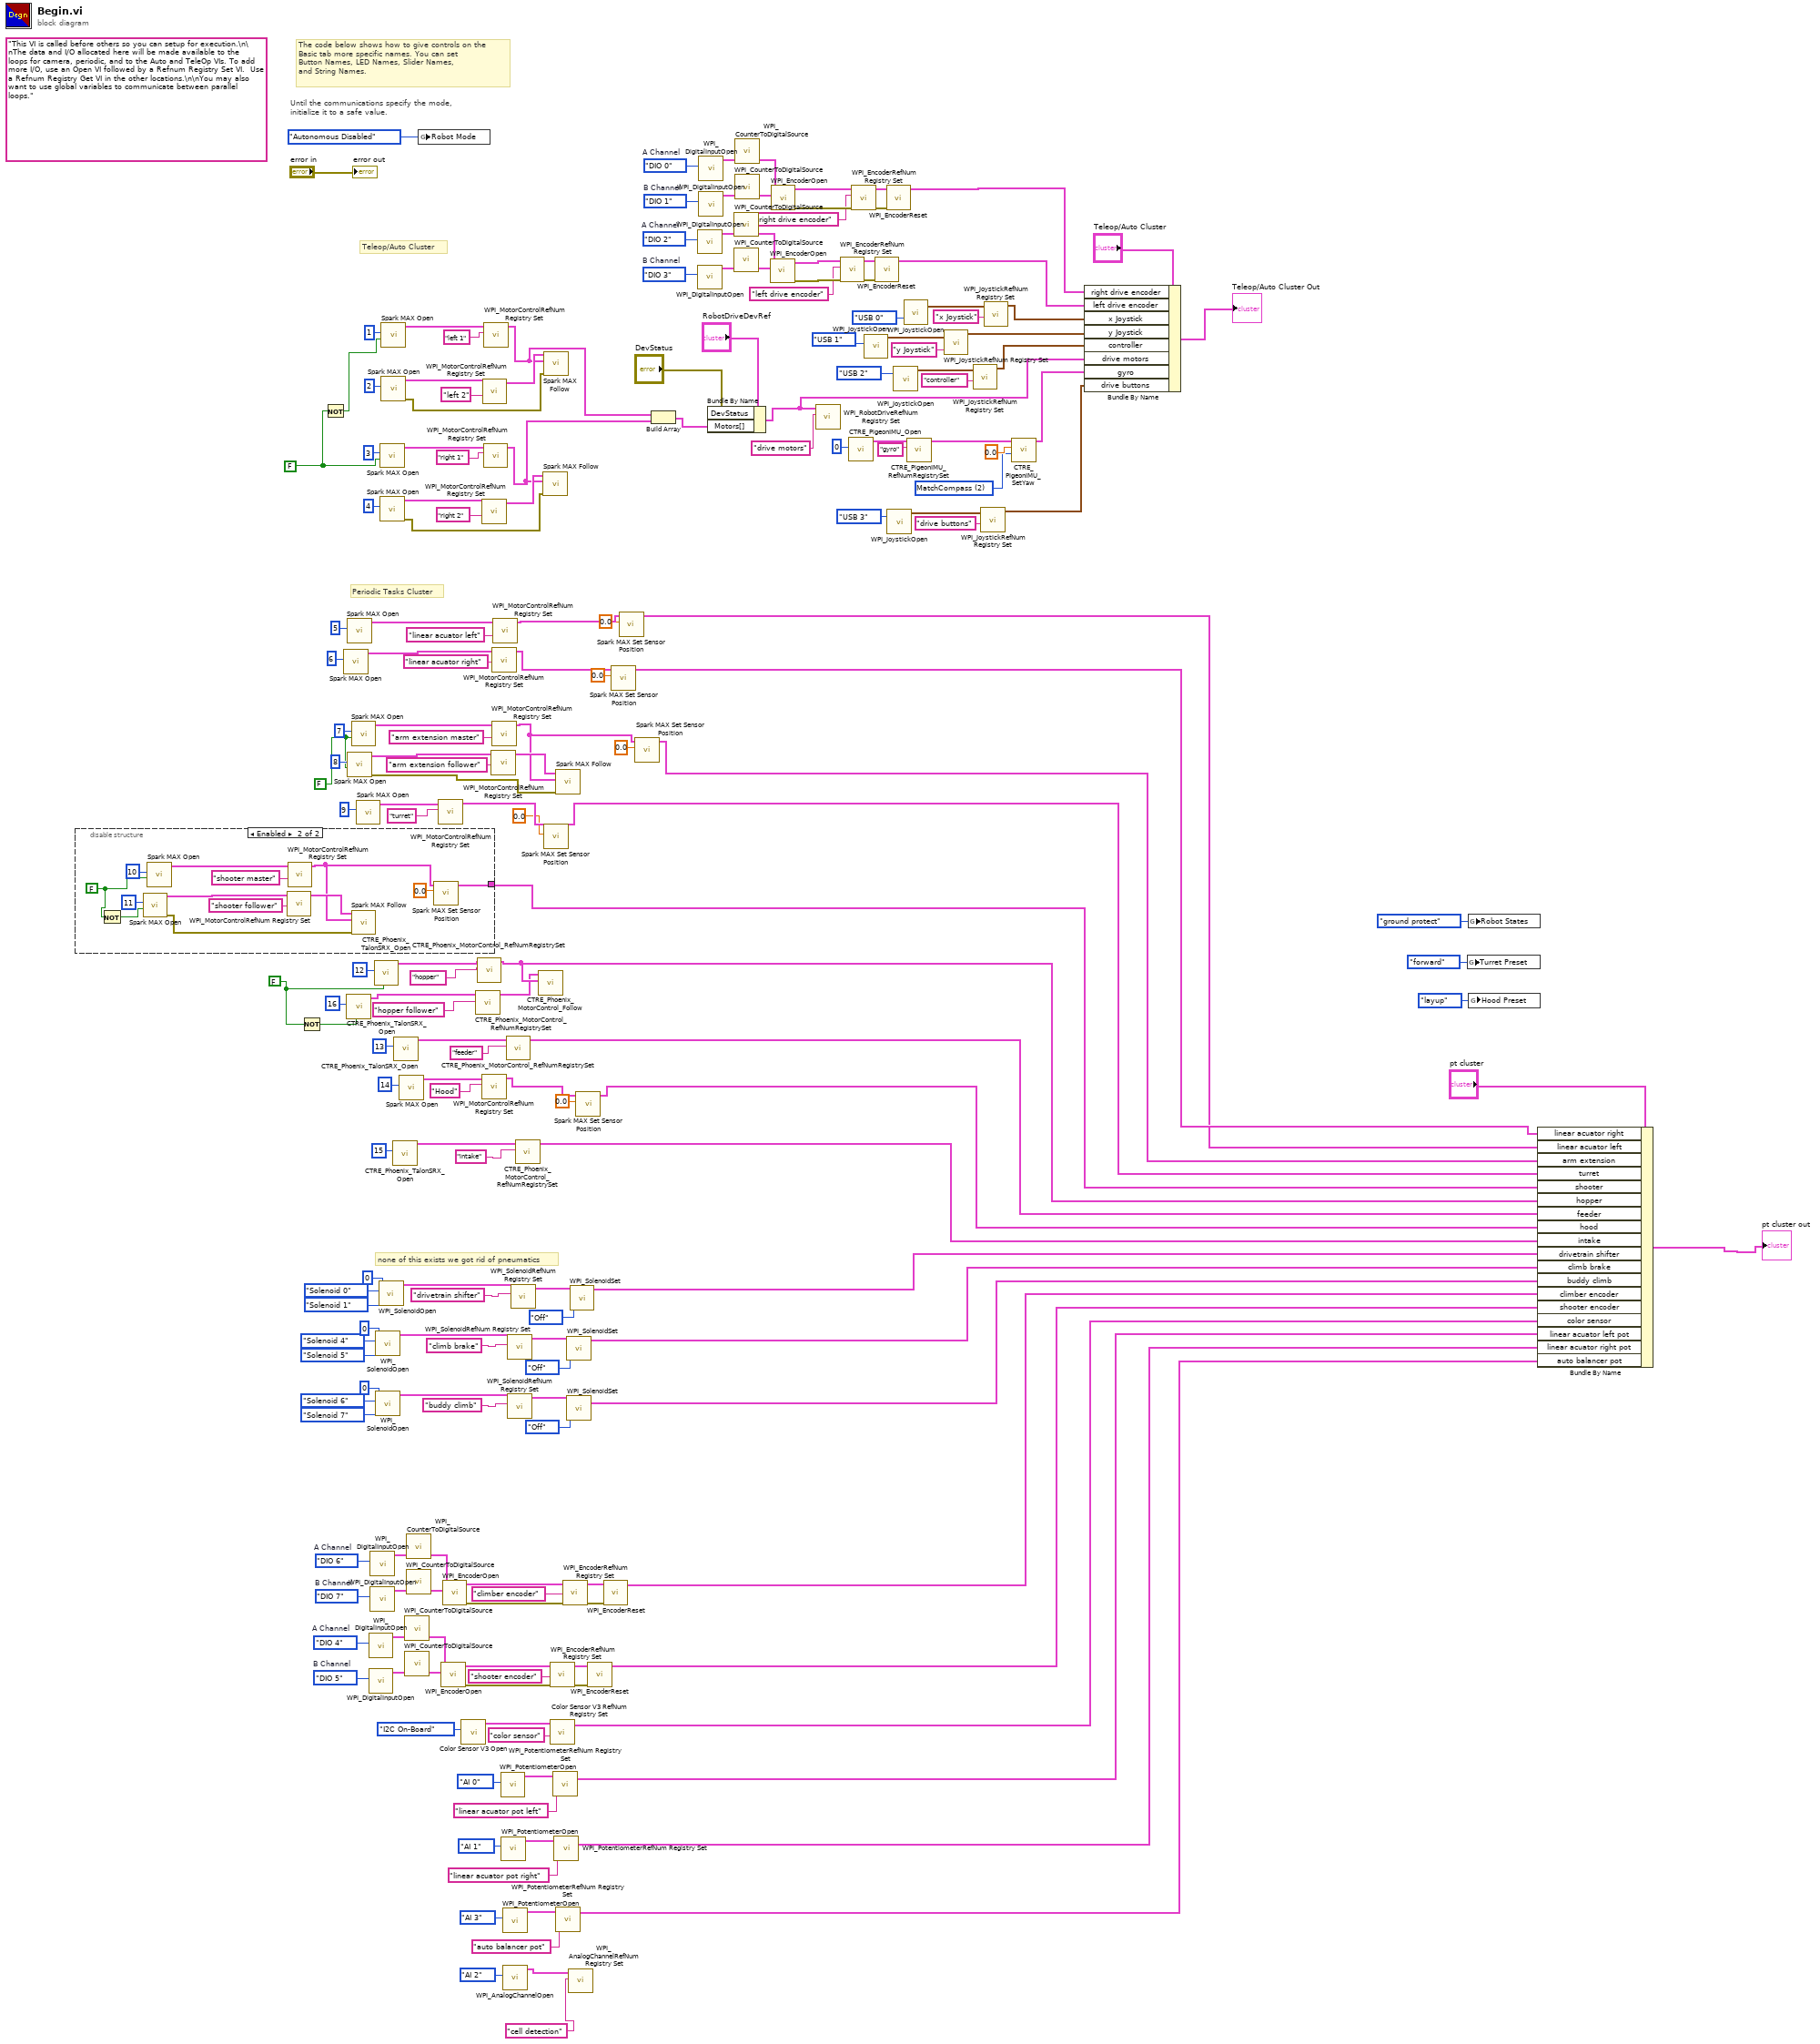
[diagram p0: block diagram]
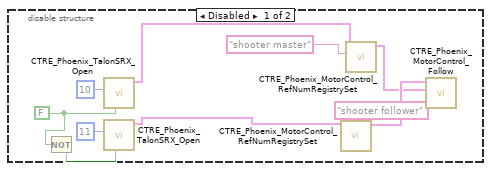
[diagram p2: hidden frame]
diagram:
  w10 = FALSE ("Invert")
  w67 = FALSE
  w89 = T26 2 items=["SetValue"=0, "AddOffset"=1, "MatchCompass"=2, "SetOffset"=255] ("TareType (SetValue)")
  w100 = FPGA_DIOChannel."DIO 5"  # B Channel
  w101 = FPGA_DIOChannel."DIO 4"  # A Channel
  w117 = FPGA_DIOChannel."DIO 7"  # B Channel
  w116 = FPGA_DIOChannel."DIO 6"  # A Channel
  w168 = FPGA_DIOChannel."DIO 3"  # B Channel
  w169 = FPGA_DIOChannel."DIO 2"  # A Channel
  w179 = FPGA_DIOChannel."DIO 1"  # B Channel
  w178 = FPGA_DIOChannel."DIO 0"  # A Channel
  w184 = FALSE
  (unwired) "This VI is called before others so you can setup for execution.\n\nThe data and I/O allocated here will be made available to the loops for camera, periodic, and to the Auto and TeleOp VIs. To add more I/O, use an Open VI followed by a Refnum Registry Set VI.  Use a Refnum Registry Get VI in the other locations.\n\nYou may also want to use global variables to communicate between parallel loops."
  # "none of this exists we got rid of pneumatics"
  # "Periodic Tasks Cluster"
  # "Teleop/Auto Cluster"
  # "The code below shows how to give controls on the\nBasic tab more specific names. You can set\nButton Names, LED Names, Slider Names,\nand String Names."
  # "Until the communications specify the mode,\ninitialize it to a safe value."
  n1 = disable-structure shown="Enabled" {
    disable-tunnel: [_ w216] -> w5
    frame Disabled {
      w206 = FALSE ("Invert")
      n2 = Not(x=w206) -> (.not. x?=w205:bool)
      n3 = call <vilib>:"CTRE_Phoenix_TalonSRX_Open.vi"("Invert"=w206, "Device Number"=u8 10) -> ("CAN Talon SRX Ref"=w208:T2)  [unwired: 8 in, 1 out]
      n4 = call <vilib>:"CTRE_Phoenix_TalonSRX_Open.vi"("Invert"=w205, "Device Number"=u8 11) -> ("CAN Talon SRX Ref"=w204:T2)  [unwired: 8 in, 1 out]
      n5 = call <vilib>:"CTRE_Phoenix_MotorControl_RefNumRegistrySet.vi"("refnum name"="shooter follower", "PhoenixMotorControlDevRef"=w204) -> ("PhoenixMotorControlDevRef"=w210:T2)  [unwired: 8 in, 1 out]
      n6 = call <vilib>:"CTRE_Phoenix_MotorControl_RefNumRegistrySet.vi"("refnum name"="shooter master", "PhoenixMotorControlDevRef"=w208) -> ("PhoenixMotorControlDevRef"=w207:T2)  [unwired: 8 in, 1 out]
      n7 = call <vilib>:"CTRE_Phoenix_MotorControl_Follow.vi"("Master Controller to Follow"=w207, "PhoenixMotorControlDevRef"=w210) -> ()  [unwired: 8 in, 2 out]
    }
    frame Enabled {
      w215 = FALSE
      n8 = Not(x=w215) -> (.not. x?=w214:bool)
      n9 = call <vilib>:"Spark MAX Open.vi"("Invert"=w214, "Device Number"=u8 11) -> ("error out"=w219:errorcluster, "MotorControlDeviceRef"=w225:T2)  [unwired: 8 in]
      n10 = call <vilib>:"Spark MAX Open.vi"("Invert"=w215, "Device Number"=u8 10) -> ("MotorControlDeviceRef"=w226:T2)  [unwired: 8 in, 1 out]
      n11 = call <vilib>:"WPI_MotorControlRefNum Registry Set.vi"("refnum name"="shooter follower", "MotorControlDevRef"=w225) -> ("MotorControlDevRef"=w224:T2)  [unwired: 8 in, 1 out]
      n12 = call <vilib>:"WPI_MotorControlRefNum Registry Set.vi"("refnum name"="shooter master", "MotorControlDevRef"=w226) -> ("MotorControlDevRef"=w217:T2)  [unwired: 8 in, 1 out]
      n13 = call <vilib>:"Spark MAX Follow.vi"("error in (no error)"=w219, "Master Controller"=w217, "MotorControlDeviceRef"=w224) -> ()  [unwired: 7 in, 2 out]
      n14 = call <vilib>:"Spark MAX Set Sensor Position.vi"("Position"=0.0, "MotorControlDeviceRef"=w217) -> ("MotorControlDeviceRef"=w216:T2)  [unwired: 8 in, 1 out]
    }
  }
  n15 = Not(x=w10) -> (.not. x?=w4:bool)
  n16 = Not(x=w184) -> (.not. x?=w185:bool)
  n17 = call <vilib>:"Spark MAX Open.vi"("Device Number"=u8 6) -> ("MotorControlDeviceRef"=w143:T2)  [unwired: 9 in, 1 out]
  n18 = call <vilib>:"CTRE_Phoenix_TalonSRX_Open.vi"("Invert"=w4, "Device Number"=u8 16) -> ("CAN Talon SRX Ref"=w11:T2)  [unwired: 8 in, 1 out]
  n19 = call <vilib>:"Spark MAX Open.vi"("Device Number"=u8 5) -> ("MotorControlDeviceRef"=w142:T2)  [unwired: 9 in, 1 out]
  n20 = call <vilib>:"Spark MAX Open.vi"("Invert"=w67, "Device Number"=u8 8) -> ("error out"=w70:errorcluster, "MotorControlDeviceRef"=w68:T2)  [unwired: 8 in]
  n21 = call <vilib>:"Spark MAX Open.vi"("Invert"=w67, "Device Number"=u8 7) -> ("MotorControlDeviceRef"=w34:T2)  [unwired: 8 in, 1 out]
  n22 = call <vilib>:"Spark MAX Open.vi"("Device Number"=u8 9) -> ("MotorControlDeviceRef"=w139:T2)  [unwired: 9 in, 1 out]
  n23 = call <vilib>:"WPI_DigitalInputOpen.vi"("DIO Channel"=w101) -> ("DigitalInputDevRef"=w104:T28)  [unwired: 1 in, 9 out]
  n24 = call <vilib>:"WPI_DigitalInputOpen.vi"("DIO Channel"=w100) -> ("DigitalInputDevRef"=w103:T28)  [unwired: 1 in, 9 out]
  n25 = call <vilib>:"WPI_DigitalInputOpen.vi"("DIO Channel"=w116) -> ("DigitalInputDevRef"=w113:T28)  [unwired: 1 in, 9 out]
  n26 = call <vilib>:"WPI_DigitalInputOpen.vi"("DIO Channel"=w117) -> ("DigitalInputDevRef"=w114:T28)  [unwired: 1 in, 9 out]
  n27 = call <vilib>:"CTRE_Phoenix_TalonSRX_Open.vi"("Invert"=w10, "Device Number"=u8 12) -> ("CAN Talon SRX Ref"=w45:T2)  [unwired: 8 in, 1 out]
  n28 = call-poly <vilib>:"WPI_SolenoidOpen.vi"("Reverse Solenoid Channel"=WPI_SolenoidChannel."Solenoid 5", "Forward Solenoid Channel"=WPI_SolenoidChannel."Solenoid 4", "Pneumatics Control Module (0)"=u8 0) -> ("SolenoidDevRef"=w121:T7)  [unwired: 7 in, 1 out]
  n29 = call-poly <vilib>:"WPI_SolenoidOpen.vi"("Reverse Solenoid Channel"=WPI_SolenoidChannel."Solenoid 7", "Forward Solenoid Channel"=WPI_SolenoidChannel."Solenoid 6", "Pneumatics Control Module (0)"=u8 0) -> ("SolenoidDevRef"=w78:T7)  [unwired: 7 in, 1 out]
  n30 = call-poly <vilib>:"WPI_SolenoidOpen.vi"("Reverse Solenoid Channel"=WPI_SolenoidChannel."Solenoid 1", "Forward Solenoid Channel"=WPI_SolenoidChannel."Solenoid 0", "Pneumatics Control Module (0)"=u8 0) -> ("SolenoidDevRef"=w128:T7)  [unwired: 7 in, 1 out]
  n31 = call <vilib>:"Spark MAX Open.vi"("Invert"=w184, "Device Number"=u8 3) -> ("MotorControlDeviceRef"=w189:T2)  [unwired: 8 in, 1 out]
  n32 = call <vilib>:"Spark MAX Open.vi"("Device Number"=u8 4) -> ("error out"=w192:errorcluster, "MotorControlDeviceRef"=w188:T2)  [unwired: 9 in]
  n33 = call <vilib>:"Spark MAX Open.vi"("Invert"=w185, "Device Number"=u8 1) -> ("MotorControlDeviceRef"=w198:T2)  [unwired: 8 in, 1 out]
  n34 = call <vilib>:"Spark MAX Open.vi"("Device Number"=u8 2) -> ("error out"=w195:errorcluster, "MotorControlDeviceRef"=w199:T2)  [unwired: 9 in]
  n35 = call <vilib>:"CTRE_Phoenix_TalonSRX_Open.vi"("Device Number"=u8 15) -> ("CAN Talon SRX Ref"=w40:T2)  [unwired: 9 in, 1 out]
  n36 = call <vilib>:"CTRE_Phoenix_TalonSRX_Open.vi"("Device Number"=u8 13) -> ("CAN Talon SRX Ref"=w42:T2)  [unwired: 9 in, 1 out]
  n37 = call <vilib>:"Spark MAX Open.vi"("Device Number"=u8 14) -> ("MotorControlDeviceRef"=w49:T2)  [unwired: 9 in, 1 out]
  n38 = call-poly <vilib>:"WPI_CounterToDigitalSource.vi"("DigitalInputDevRef"=w104) -> ("Digital Source"=w105:T29)  [unwired: 6 out]
  n39 = call-poly <vilib>:"WPI_CounterToDigitalSource.vi"("DigitalInputDevRef"=w103) -> ("Digital Source"=w102:T29)  [unwired: 6 out]
  n40 = call-poly <vilib>:"WPI_CounterToDigitalSource.vi"("DigitalInputDevRef"=w113) -> ("Digital Source"=w112:T29)  [unwired: 6 out]
  n41 = call-poly <vilib>:"WPI_CounterToDigitalSource.vi"("DigitalInputDevRef"=w114) -> ("Digital Source"=w115:T29)  [unwired: 6 out]
  n42 = global write "Robot Global Data.vi" "Robot Mode"(WPI_DriverStationRobotMode2."Autonomous Disabled" ("Robot Mode")) -> ()
  n43 = call <vilib>:"WPI_MotorControlRefNum Registry Set.vi"("refnum name"="turret", "MotorControlDevRef"=w139) -> ("MotorControlDevRef"=w20:T2)  [unwired: 8 in, 1 out]
  n44 = call <vilib>:"WPI_EncoderOpen.vi"("BSource"=w102, "ASource"=w105) -> ("error out"=w106:errorcluster, "EncoderDevRef"=w107:T9)  [unwired: 6 in, 2 out]
  n45 = call <vilib>:"WPI_EncoderOpen.vi"("BSource"=w115, "ASource"=w112) -> ("error out"=w111:errorcluster, "EncoderDevRef"=w110:T9)  [unwired: 6 in, 2 out]
  n46 = call <vilib>:"Color Sensor V3 Open.vi"("I2C Bus"=i2c_bus."I2C On-Board") -> ("ColorSensorDevRef"=w96:T13)  [unwired: 9 in, 1 out]
  n47 = call <vilib>:"CTRE_Phoenix_MotorControl_RefNumRegistrySet.vi"("refnum name"="hopper follower", "PhoenixMotorControlDevRef"=w11) -> ("PhoenixMotorControlDevRef"=w12:T2)  [unwired: 8 in, 1 out]
  n48 = call <vilib>:"CTRE_Phoenix_MotorControl_RefNumRegistrySet.vi"("refnum name"="hopper", "PhoenixMotorControlDevRef"=w45) -> ("PhoenixMotorControlDevRef"=w13:T2)  [unwired: 8 in, 1 out]
  n49 = call <vilib>:"WPI_MotorControlRefNum Registry Set.vi"("refnum name"="right 2", "MotorControlDevRef"=w188) -> ("MotorControlDevRef"=w191:T2)  [unwired: 8 in, 1 out]
  n50 = call <vilib>:"WPI_MotorControlRefNum Registry Set.vi"("refnum name"="Hood", "MotorControlDevRef"=w49) -> ("MotorControlDevRef"=w18:T2)  [unwired: 8 in, 1 out]
  n51 = call <vilib>:"WPI_MotorControlRefNum Registry Set.vi"("refnum name"="left 2", "MotorControlDevRef"=w199) -> ("MotorControlDevRef"=w196:T2)  [unwired: 8 in, 1 out]
  n52 = call <vilib>:"WPI_MotorControlRefNum Registry Set.vi"("refnum name"="right 1", "MotorControlDevRef"=w189) -> ("MotorControlDevRef"=w37:T2)  [unwired: 8 in, 1 out]
  n53 = call <vilib>:"WPI_MotorControlRefNum Registry Set.vi"("refnum name"="left 1", "MotorControlDevRef"=w198) -> ("MotorControlDevRef"=w36:T2)  [unwired: 8 in, 1 out]
  n54 = call <vilib>:"WPI_MotorControlRefNum Registry Set.vi"("refnum name"="arm extension follower", "MotorControlDevRef"=w68) -> ("MotorControlDevRef"=w69:T2)  [unwired: 8 in, 1 out]
  n55 = call <vilib>:"WPI_MotorControlRefNum Registry Set.vi"("refnum name"="linear acuator right", "MotorControlDevRef"=w143) -> ("MotorControlDevRef"=w29:T2)  [unwired: 8 in, 1 out]
  n56 = call <vilib>:"WPI_MotorControlRefNum Registry Set.vi"("refnum name"="arm extension master", "MotorControlDevRef"=w34) -> ("MotorControlDevRef"=w33:T2)  [unwired: 8 in, 1 out]
  n57 = call <vilib>:"WPI_MotorControlRefNum Registry Set.vi"("refnum name"="linear acuator left", "MotorControlDevRef"=w142) -> ("MotorControlDevRef"=w31:T2)  [unwired: 8 in, 1 out]
  n58 = call <vilib>:"WPI_PotentiometerOpen.vi"("Analog Channel"=FPGA_AIChannel."AI 0") -> ("PotDevRef"=w62:T16)  [unwired: 9 in, 1 out]
  n59 = call <vilib>:"WPI_PotentiometerOpen.vi"("Analog Channel"=FPGA_AIChannel."AI 1") -> ("PotDevRef"=w65:T16)  [unwired: 9 in, 1 out]
  n60 = call <vilib>:"WPI_PotentiometerOpen.vi"("Analog Channel"=FPGA_AIChannel."AI 3") -> ("PotDevRef"=w59:T16)  [unwired: 9 in, 1 out]
  n61 = call <vilib>:"WPI_AnalogChannelOpen.vi"("Analog Channel"=FPGA_AIChannel."AI 2") -> ("AIDeviceRef"=w2:T33)  [unwired: 9 in, 1 out]
  n62 = call <vilib>:"CTRE_Phoenix_MotorControl_RefNumRegistrySet.vi"("refnum name"="feeder", "PhoenixMotorControlDevRef"=w42) -> ("PhoenixMotorControlDevRef"=w41:T2)  [unwired: 8 in, 1 out]
  n63 = call <vilib>:"WPI_SolenoidRefNum Registry Set.vi"("refnum name"="climb brake", "SolenoidDevRef"=w121) -> ("SolenoidDevRef"=w119:T7)  [unwired: 8 in, 1 out]
  n64 = call <vilib>:"WPI_SolenoidRefNum Registry Set.vi"("refnum name"="buddy climb", "SolenoidDevRef"=w78) -> ("SolenoidDevRef"=w80:T7)  [unwired: 8 in, 1 out]
  n65 = call <vilib>:"WPI_SolenoidRefNum Registry Set.vi"("refnum name"="drivetrain shifter", "SolenoidDevRef"=w128) -> ("SolenoidDevRef"=w126:T7)  [unwired: 8 in, 1 out]
  n66 = call <vilib>:"CTRE_Phoenix_MotorControl_RefNumRegistrySet.vi"("refnum name"="intake", "PhoenixMotorControlDevRef"=w40) -> ("PhoenixMotorControlDevRef"=w39:T2)  [unwired: 8 in, 1 out]
  n67 = call <vilib>:"CTRE_Phoenix_MotorControl_Follow.vi"("Master Controller to Follow"=w13, "PhoenixMotorControlDevRef"=w12) -> ()  [unwired: 8 in, 2 out]
  n68 = call <vilib>:"Spark MAX Follow.vi"("error in (no error)"=w192, "Master Controller"=w37, "MotorControlDeviceRef"=w191) -> ()  [unwired: 7 in, 2 out]
  n69 = call <vilib>:"Spark MAX Follow.vi"("error in (no error)"=w195, "Master Controller"=w36, "MotorControlDeviceRef"=w196) -> ()  [unwired: 7 in, 2 out]
  n70 = call <vilib>:"Spark MAX Set Sensor Position.vi"("Position"=0.0, "MotorControlDeviceRef"=w20) -> ("MotorControlDeviceRef"=w19:T2)  [unwired: 8 in, 1 out]
  n71 = call <vilib>:"WPI_EncoderRefNum Registry Set.vi"("error in (no error)"=w106, "refnum name"="shooter encoder", "EncoderDevRef"=w107) -> ("error out"=w23:errorcluster, "EncoderDevRef"=w22:T9)  [unwired: 7 in]
  n72 = call <vilib>:"Color Sensor V3 RefNum Registry Set.vi"("refnum name"="color sensor", "ColorSensorDevRef"=w96) -> ("ColorSensorDevRef out"=w50:T13)  [unwired: 8 in, 1 out]
  n73 = call <vilib>:"WPI_PotentiometerRefNum Registry Set.vi"("refnum name"="linear acuator pot left", "PotDevRef"=w62) -> ("PotDevRef"=w53:T16)  [unwired: 8 in, 1 out]
  n74 = call <vilib>:"WPI_PotentiometerRefNum Registry Set.vi"("refnum name"="linear acuator pot right", "PotDevRef"=w65) -> ("PotDevRef"=w52:T16)  [unwired: 8 in, 1 out]
  n75 = call <vilib>:"Spark MAX Follow.vi"("error in (no error)"=w70, "Master Controller"=w33, "MotorControlDeviceRef"=w69) -> ()  [unwired: 7 in, 2 out]
  n76 = call <vilib>:"WPI_PotentiometerRefNum Registry Set.vi"("refnum name"="auto balancer pot", "PotDevRef"=w59) -> ("PotDevRef"=w51:T16)  [unwired: 8 in, 1 out]
  n77 = call <vilib>:"WPI_EncoderRefNum Registry Set.vi"("error in (no error)"=w111, "refnum name"="climber encoder", "EncoderDevRef"=w110) -> ("error out"=w109:errorcluster, "EncoderDevRef"=w108:T9)  [unwired: 7 in]
  n78 = call-poly <vilib>:"WPI_SolenoidSet.vi"("Value"=WPI_SolenoidValue."Off", "SolenoidDevRef"=w119) -> ("SolenoidDevRef"=w56:T7)  [unwired: 8 in, 1 out]
  n79 = call-poly <vilib>:"WPI_SolenoidSet.vi"("Value"=WPI_SolenoidValue."Off", "SolenoidDevRef"=w80) -> ("SolenoidDevRef"=w55:T7)  [unwired: 8 in, 1 out]
  n80 = call <vilib>:"WPI_AnalogChannelRefNum Registry Set.vi"("refnum name"="cell detection", "AIDeviceRef"=w2) -> ()  [unwired: 8 in, 2 out]
  n81 = call-poly <vilib>:"WPI_SolenoidSet.vi"("Value"=WPI_SolenoidValue."Off", "SolenoidDevRef"=w126) -> ("SolenoidDevRef"=w57:T7)  [unwired: 8 in, 1 out]
  n82 = call <vilib>:"Spark MAX Set Sensor Position.vi"("Position"=0.0, "MotorControlDeviceRef"=w18) -> ("MotorControlDeviceRef"=w17:T2)  [unwired: 8 in, 1 out]
  n83 = call <vilib>:"WPI_EncoderReset.vi"("error in (no error)"=w23, "EncoderDevRef"=w22) -> ("EncoderDevRef"=w21:T9)  [unwired: 8 in, 1 out]
  n84 = call <vilib>:"WPI_EncoderReset.vi"("error in (no error)"=w109, "EncoderDevRef"=w108) -> ("EncoderDevRef"=w54:T9)  [unwired: 8 in, 1 out]
  n85 = call <vilib>:"Spark MAX Set Sensor Position.vi"("Position"=0.0, "MotorControlDeviceRef"=w29) -> ("MotorControlDeviceRef"=w26:T2)  [unwired: 8 in, 1 out]
  n86 = call <vilib>:"Spark MAX Set Sensor Position.vi"("Position"=0.0, "MotorControlDeviceRef"=w31) -> ("MotorControlDeviceRef"=w25:T2)  [unwired: 8 in, 1 out]
  n87 = call <vilib>:"Spark MAX Set Sensor Position.vi"("Position"=0.0, "MotorControlDeviceRef"=w33) -> ("MotorControlDeviceRef"=w32:T2)  [unwired: 8 in, 1 out]
  n88 = Build Array(w36, w37) -> (w181:T2[])
  n89 = call <vilib>:"WPI_DigitalInputOpen.vi"("DIO Channel"=w169) -> ("DigitalInputDevRef"=w172:T28)  [unwired: 1 in, 9 out]
  n90 = call <vilib>:"WPI_DigitalInputOpen.vi"("DIO Channel"=w168) -> ("DigitalInputDevRef"=w171:T28)  [unwired: 1 in, 9 out]
  n91 = call <vilib>:"WPI_DigitalInputOpen.vi"("DIO Channel"=w178) -> ("DigitalInputDevRef"=w175:T28)  [unwired: 1 in, 9 out]
  n92 = call <vilib>:"WPI_DigitalInputOpen.vi"("DIO Channel"=w179) -> ("DigitalInputDevRef"=w176:T28)  [unwired: 1 in, 9 out]
  n93 = Bundle By Name(cluster="RobotDriveDevRef", "DevStatus"="DevStatus", "Motors[]"=w181) -> (w46:T21)
  n94 = call-poly <vilib>:"WPI_CounterToDigitalSource.vi"("DigitalInputDevRef"=w172) -> ("Digital Source"=w173:T29)  [unwired: 6 out]
  n95 = call-poly <vilib>:"WPI_CounterToDigitalSource.vi"("DigitalInputDevRef"=w171) -> ("Digital Source"=w170:T29)  [unwired: 6 out]
  n96 = call-poly <vilib>:"WPI_CounterToDigitalSource.vi"("DigitalInputDevRef"=w175) -> ("Digital Source"=w174:T29)  [unwired: 6 out]
  n97 = call-poly <vilib>:"WPI_CounterToDigitalSource.vi"("DigitalInputDevRef"=w176) -> ("Digital Source"=w177:T29)  [unwired: 6 out]
  n98 = call <vilib>:"WPI_EncoderOpen.vi"("BSource"=w170, "ASource"=w173) -> ("error out"=w162:errorcluster, "EncoderDevRef"=w167:T9)  [unwired: 6 in, 2 out]
  n99 = call <vilib>:"WPI_EncoderOpen.vi"("BSource"=w177, "ASource"=w174) -> ("error out"=w163:errorcluster, "EncoderDevRef"=w166:T9)  [unwired: 6 in, 2 out]
  n100 = call <vilib>:"WPI_RobotDriveRefNum Registry Set.vi"("refnum name"="drive motors", "RobotDriveDevRef"=w46) -> ()  [unwired: 8 in, 2 out]
  n101 = call <vilib>:"WPI_EncoderRefNum Registry Set.vi"("error in (no error)"=w162, "refnum name"="left drive encoder", "EncoderDevRef"=w167) -> ("error out"=w161:errorcluster, "EncoderDevRef"=w160:T9)  [unwired: 7 in]
  n102 = call-poly <vilib>:"CTRE_PigeonIMU_Open.vi"("Device Number"=u8 0) -> ("PigeonIMUDevRef"=w94:T22)  [unwired: 9 in, 1 out]
  n103 = call <vilib>:"WPI_EncoderRefNum Registry Set.vi"("error in (no error)"=w163, "refnum name"="right drive encoder", "EncoderDevRef"=w166) -> ("error out"=w165:errorcluster, "EncoderDevRef"=w164:T9)  [unwired: 7 in]
  n104 = call <vilib>:"WPI_JoystickOpen.vi"("JoystickDevice"=WPI_JoystickDeviceEnum."USB 1") -> ("JoystickDevRef"=w153:T19)  [unwired: 10 in]
  n105 = call <vilib>:"WPI_EncoderReset.vi"("error in (no error)"=w161, "EncoderDevRef"=w160) -> ("EncoderDevRef"=w147:T9)  [unwired: 8 in, 1 out]
  n106 = call <vilib>:"WPI_EncoderReset.vi"("error in (no error)"=w165, "EncoderDevRef"=w164) -> ("EncoderDevRef"=w148:T9)  [unwired: 8 in, 1 out]
  n107 = call <vilib>:"WPI_JoystickOpen.vi"("JoystickDevice"=WPI_JoystickDeviceEnum."USB 3") -> ("JoystickDevRef"=w84:T19)  [unwired: 10 in]
  n108 = call <vilib>:"WPI_JoystickOpen.vi"("JoystickDevice"=WPI_JoystickDeviceEnum."USB 2") -> ("JoystickDevRef"=w154:T19)  [unwired: 10 in]
  n109 = call <vilib>:"WPI_JoystickOpen.vi"("JoystickDevice"=WPI_JoystickDeviceEnum."USB 0") -> ("JoystickDevRef"=w152:T19)  [unwired: 10 in]
  n110 = call <vilib>:"CTRE_PigeonIMU_RefNumRegistrySet.vi"("refnum name"="gyro", "PigeonIMUDevRef"=w94) -> ("PigeonIMUDevRef"=w91:T22)  [unwired: 8 in, 1 out]
  n111 = call <vilib>:"WPI_JoystickRefNum Registry Set.vi"("refnum name"="y Joystick", "JoystickDevRef"=w153) -> ("JoystickDevRef"=w145:T19)  [unwired: 8 in, 1 out]
  n112 = call <vilib>:"WPI_JoystickRefNum Registry Set.vi"("refnum name"="controller", "JoystickDevRef"=w154) -> ("JoystickDevRef"=w146:T19)  [unwired: 8 in, 1 out]
  n113 = call <vilib>:"WPI_JoystickRefNum Registry Set.vi"("refnum name"="drive buttons", "JoystickDevRef"=w84) -> ("JoystickDevRef"=w82:T19)  [unwired: 8 in, 1 out]
  n114 = call <vilib>:"WPI_JoystickRefNum Registry Set.vi"("refnum name"="x Joystick", "JoystickDevRef"=w152) -> ("JoystickDevRef"=w144:T19)  [unwired: 8 in, 1 out]
  n115 = call <vilib>:"CTRE_PigeonIMU_SetYaw.vi"("TareType (SetValue)"=w89, "Value"=0.0, "PigeonIMUDevRef"=w91) -> ("PigeonIMUDevRef"=w88:T22)  [unwired: 7 in, 1 out]
  n116 = Bundle By Name(cluster="Teleop/Auto Cluster", "right drive encoder"=w148, "left drive encoder"=w147, "x Joystick"=w144, "y Joystick"=w145, "controller"=w146, "drive motors"=w46, "gyro"=w88, "drive buttons"=w82) -> (→"Teleop/Auto Cluster Out":T18)
  n117 = global write "GlobalVariables.vi" "Turret Preset"(enum16{"free track", "forward", "backward"}."forward" ("Turret Preset")) -> ()
  n118 = global write "GlobalVariables.vi" "Robot States"(T24."ground protect" ("Robot States")) -> ()
  n119 = global write "GlobalVariables.vi" "Hood Preset"(enum16{"trench", "layup", "free track"}."layup" ("Hood Preset")) -> ()
  n120 = Bundle By Name(cluster="pt cluster", "linear acuator right"=w26, "linear acuator left"=w25, "arm extension"=w32, "turret"=w19, "shooter"=w5, "hopper"=w13, "feeder"=w41, "hood"=w17, "intake"=w39, "drivetrain shifter"=w57, "climb brake"=w56, "buddy climb"=w55, "climber encoder"=w54, "shooter encoder"=w21, "color sensor"=w50, "linear acuator left pot"=w53, "linear acuator right pot"=w52, "auto balancer pot"=w51) -> (→"pt cluster out":T1)
  "error out" <- "error in"
